vi "Try Match Response.vi"(8 "error in":errorcluster, 10 "ICAN CC Frame":refnum<class "ICAN CC Frame.lvclass">, 11 "Expedited Download Transfer in":refnum<class "Expedited Download Transfer.lvclass">) -> (0 "error out":errorcluster, 2 "Match":bool, 3 "Expedited Download Transfer out":refnum<class "SDO Transfer.lvclass">)   [LabVIEW 2020, in "CANopen.lvlib" / "SDO Manager.lvlib" / "Expedited Download Transfer.lvclass"]
uses:
  Expedited Download Transfer.lvclass
  SDO Transfer/SDO Transfer.lvclass
  HAL/Source/Interfaces/ICAN CC Frame/ICAN CC Frame.lvclass
  Expedited Download Transfer.lvclass/Expedited Download Transfer.ctl
  Typedefs/SDO Result.ctl
  SDO Transfer/SDO abort code.ctl
  CANopen Message/CANopen Message.lvclass
  SDO Transfer/SDO Transfer Result.ctl
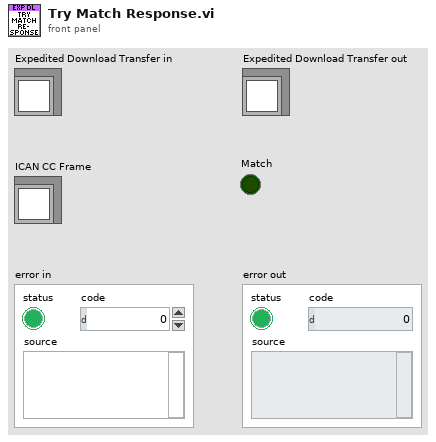
[diagram p1: front panel]
types:
  T1 = typedef "CANopen.lvlib/SDO Manager.lvlib/SDO Transfer.lvclass/SDO Transfer Result.ctl" = cluster{"SDO Result":T2, "Error":errorcluster}
  T2 = typedef "CANopen.lvlib/SDO Manager.lvlib/SDO Transfer.lvclass/SDO Result.ctl" = cluster{"Success":bool, "SDO abort code":cluster{"Null":bool, "Value":T3}, "Data":cluster{"Null":bool, "Data":u8[]}}
  T3 = typedef "CANopen.lvlib/SDO Manager.lvlib/SDO Transfer.lvclass/SDO abort code.ctl" = u32
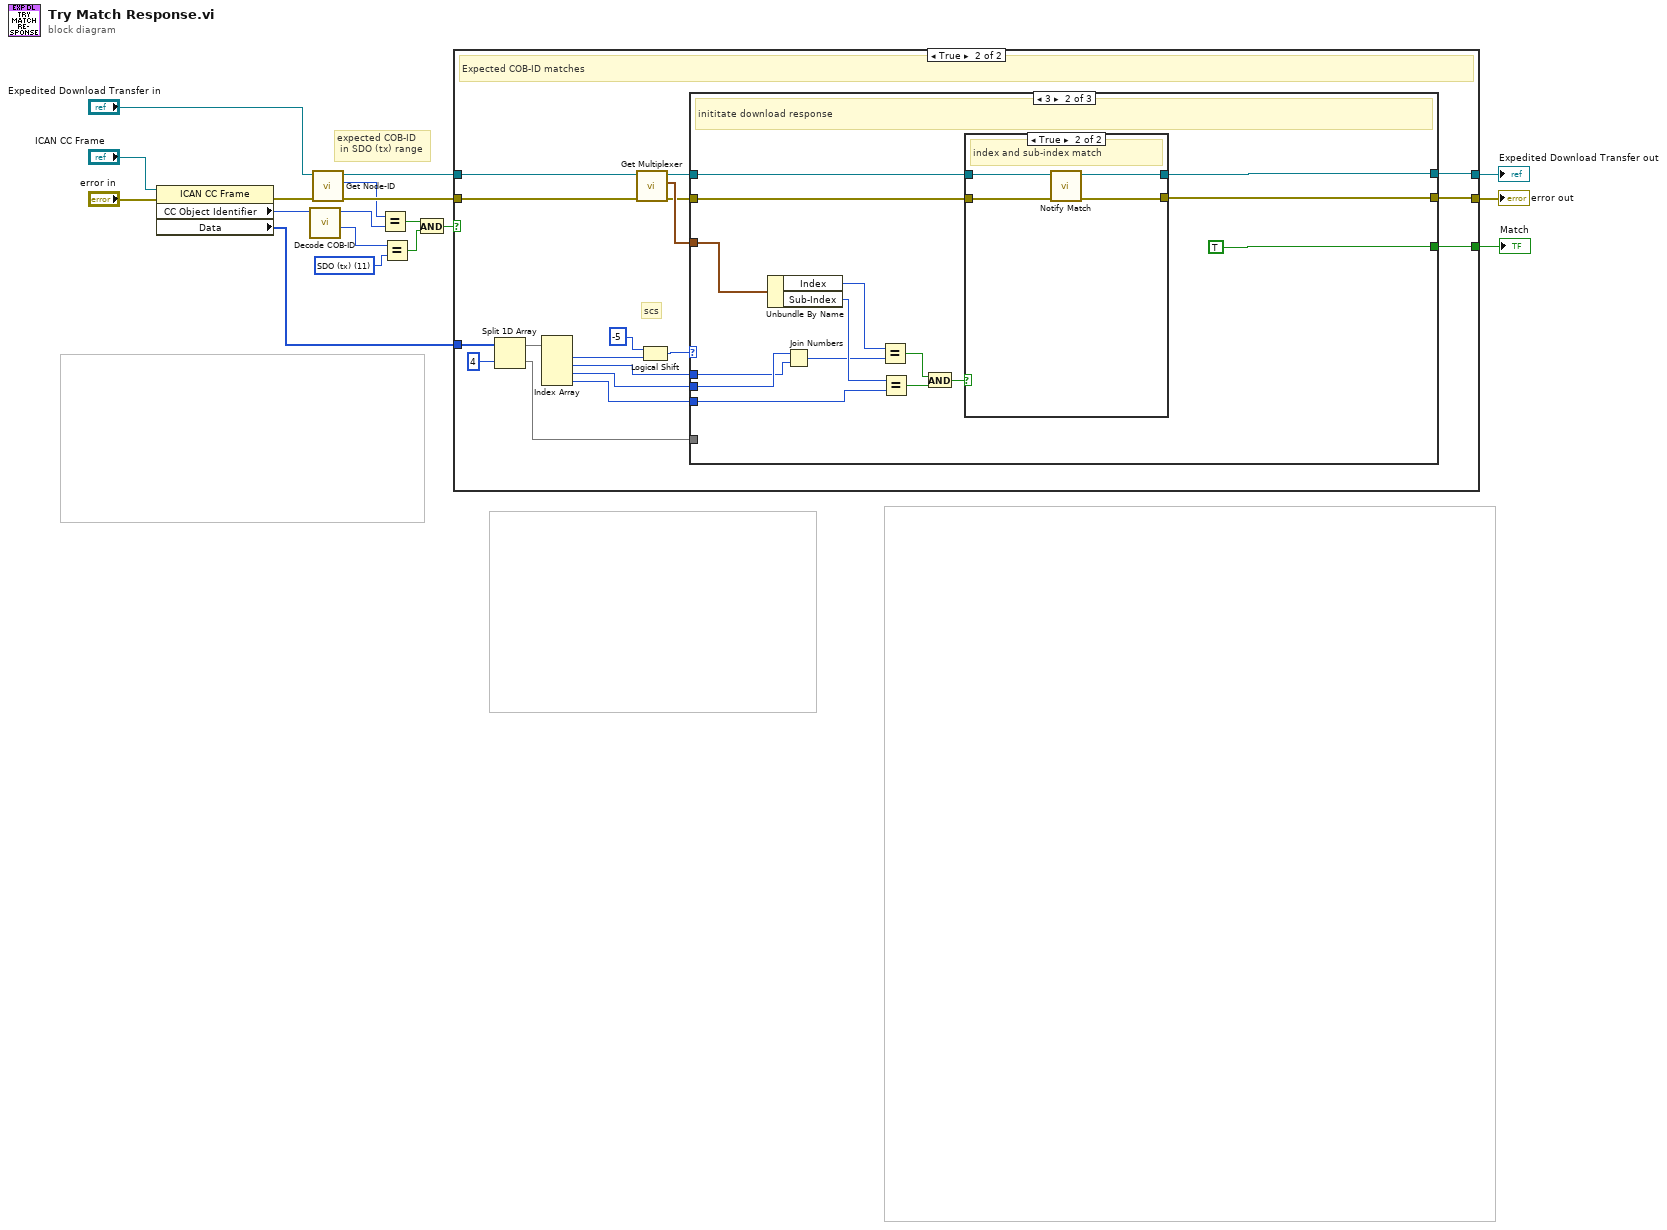
[diagram p0: block diagram]
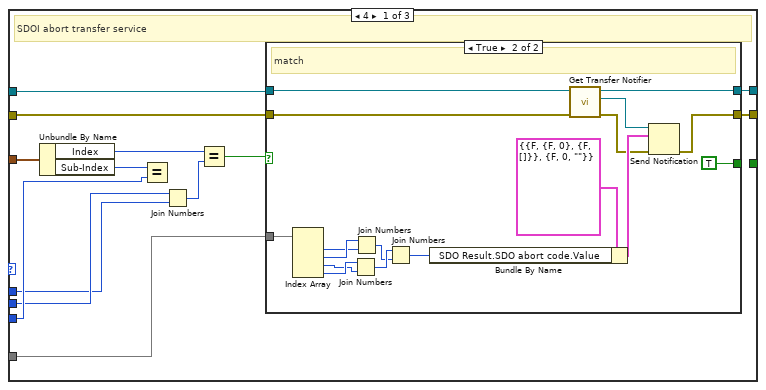
[diagram p3: hidden frame]
diagram:
  w3 = u8 11 items=["NMT"=0, "EMCY/SYNC"=1, "TIME"=2, "PDO1 (tx)"=3, "PDO1 (rx)"=4, "PDO2 (tx)"=5, "PDO2 (rx)"=6, "PDO3 (tx)"=7, "PDO3 (rx)"=8, "PDO4 (tx)"=9, "PDO4 (rx)"=10, "SDO (tx)"=11, "SDO (rx)"=12, "NMT error control"=14] ("Function Code")
  # "expected COB-ID\n in SDO (tx) range"
  n1 = property class="ICAN CC Frame"(reference="ICAN CC Frame", error in="error in") -> (error out=w16:errorcluster, "CC Object Identifier"=w7:u32, "Data"=w9:u8[])  [unwired: 1 out]
  n2 = call "Decode COB-ID.vi"("COD-ID"=w7) -> ("Function Code"=w2:u8, "Node-ID"=w6:u8)  [unwired: 9 in]
  n3 = call "Get Node-ID.vi"("error in"=w16, "SDO Transfer in"="Expedited Download Transfer in") -> ("error out"=w13:errorcluster, "Node-ID"=w5:u8, "SDO Transfer out"=w14:refnum<class "Expedited Download Transfer.lvclass">)  [unwired: 7 in]
  n4 = Equal?(x=w5, y=w6) -> (x = y?=w12:bool)
  n5 = Equal?(x=w2, y=w3) -> (x = y?=w1:bool)
  n6 = And(x=w12, y=w1) -> (x .and. y?=w4:bool)
  n7 = case shown="True" w4 {
    tunnel: w14 -> [w20 w36]
    tunnel: w13 -> [w19 w35]
    tunnel: [w20 w26] -> w11
    tunnel: [w19 w27] -> w10
    tunnel: w9 -> [_ w23]
    tunnel: [_ w25] -> w8
    frame False {
    }
    frame True {
      # "scs"
      # "Expected COB-ID matches"
      n8 = Split 1D Array(array=w23, index=4) -> (first subarray=w22:u8[], second subarray=w21:u8[])
      n9 = Index Array(array=w22) -> (element #1=w38:u8, element #2=w32:u8, element #3=w31:u8, element #4=w30:u8)  [unwired: 4 in]
      n10 = call "Get Multiplexer.vi"("error in"=w35, "SDO Transfer in"=w36) -> ("error out"=w28:errorcluster, "Multiplexer"=w33:cluster{"Index":u16, "Sub-Index":u8}, "SDO Transfer out"=w29:refnum<class "Expedited Download Transfer.lvclass">)  [unwired: 7 in]
      n11 = Logical Shift(y=i16 -5, x=w38) -> (x << y=w34:u8)
      n12 = case shown="3" w34 {
        tunnel: w33 -> [w47 w82 _]
        tunnel: w32 -> [w44 w78 _]
        tunnel: w31 -> [w45 w79 _]
        tunnel: w30 -> [w46 w77 _]
        tunnel: w29 -> [w51 w74 w92]
        tunnel: w28 -> [w39 w76 w93]
        tunnel: [w40 w73 w92] -> w26
        tunnel: [w41 w75 w93] -> w27
        tunnel: [_ TRUE _] -> w25
        tunnel: w21 -> [w42 _ _]
        frame 4 {
          # "SDOI abort transfer service"
          n13 = Unbundle By Name(w47) -> ("Index"=w50:u16, "Sub-Index"=w49:u8)
          n14 = Equal?(x=w49, y=w46) -> ()  [unwired: 1 out]
          n15 = Join Numbers(hi=w45, lo=w44) -> ((hi.lo)=w48:u16)
          n16 = Equal?(x=w50, y=w48) -> (x = y?=w43:bool)
          n17 = case shown="True" w43 {
            tunnel: w51 -> [w53 w68]
            tunnel: [w53 w66] -> w40
            tunnel: [w52 w62] -> w41
            tunnel: [_ TRUE] -> _
            tunnel: w42 -> [_ w60]
            tunnel: w39 -> [w52 w55]
            frame False {
              # "no match"
            }
            frame True {
              # "match"
              n18 = Index Array(array=w60) -> (element #1=w58:u8, element #2=w59:u8, element #3=w56:u8, element #4=w57:u8)  [unwired: 4 in]
              n19 = Join Numbers(hi=w57, lo=w56) -> ((hi.lo)=w70:u16)
              n20 = Join Numbers(hi=w59, lo=w58) -> ((hi.lo)=w69:u16)
              n21 = Join Numbers(hi=w70, lo=w69) -> ((hi.lo)=w64:u32)
              n22 = Bundle By Name(cluster=T1 {"SDO Result"={"Success"=FALSE, "SDO abort code"={"Null"=FALSE, "Value"=0}, "Data"={"Null"=FALSE, "Data"=[]}}, "Error"={"status"=FALSE, "code"=0, "source"=""}} ("SDO Transfer Result"), "SDO Result.SDO abort code.Value"=w64) -> (w65:T1)
              n23 = call "Get Transfer Notifier.vi"("error in"=w55, "SDO Transfer in"=w68) -> ("error out"=w63:errorcluster, "SDO Transfer Notifier"=w67:refnum<notifier>, "SDO Transfer out"=w66:refnum<class "Expedited Download Transfer.lvclass">)  [unwired: 7 in]
              n24 = Send Notification(notification=w65, notifier=w67, error in (no error)=w63) -> (error out=w62:errorcluster)  [unwired: 1 out]
            }
          }
        }
        frame 3 {
          # "inititate download response"
          n25 = Unbundle By Name(w82) -> ("Index"=w83:u16, "Sub-Index"=w85:u8)
          n26 = Join Numbers(hi=w79, lo=w78) -> ((hi.lo)=w84:u16)
          n27 = Equal?(x=w83, y=w84) -> (x = y?=w81:bool)
          n28 = Equal?(x=w85, y=w77) -> (x = y?=w80:bool)
          n29 = And(x=w81, y=w80) -> (x .and. y?=w72:bool)
          n30 = case shown="True" w72 {
            tunnel: w76 -> [w87 w91]
            tunnel: [w87 w90] -> w75
            tunnel: w74 -> [w86 w89]
            tunnel: [w86 w88] -> w73
            frame False {
              # "index or sub-index no match"
            }
            frame True {
              # "index and sub-index match"
              n31 = call "Notify Match.vi"("error in"=w91, "SDO Transfer in"=w89) -> ("error out"=w90:errorcluster, "SDO Transfer out"=w88:refnum<class "Expedited Download Transfer.lvclass">)  [unwired: 8 in]
            }
          }
        }
        frame Default {
          # "scs no match"
        }
      }
    }
  }
  "Expedited Download Transfer out" <- w11
  "error out" <- w10
  "Match" <- w8
